vi "Launcher.vi"   [LabVIEW 2020]
uses:
  Executive/Executive/Executive.lvclass
  C:/Program Files (x86)/National Instruments/LabVIEW 2020/vi.lib/ActorFramework/Actor/Actor.lvclass
  <vilib>/ActorFramework/Actor/Actor.lvclass
panel:
  # "open_cst"
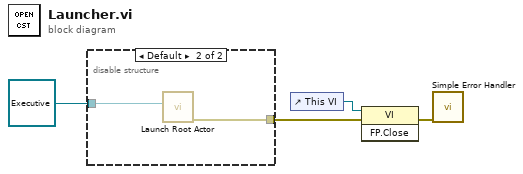
[diagram p0: block diagram]
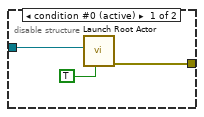
[diagram p2: hidden frame]
diagram:
  n1 = disable-structure shown="Default" {
    disable-tunnel: refnum<class "Executive.lvclass"> refnum ("Executive.lvlib:Executive.lvclass") -> [w7 w9]
    disable-tunnel: [w6 w8] -> w2
    frame condition #0 (active) {
      n2 = call <vilib>:"Launch Root Actor.vi"("Open Actor Core front panel? (F)"=TRUE, "Actor"=w7) -> ("error out"=w6:errorcluster)  [unwired: 8 in, 1 out]
    }
    frame condition #1 {
      n3 = call <vilib>:"Launch Root Actor.vi"("Actor"=w9) -> ("error out"=w8:errorcluster)  [unwired: 9 in, 1 out]
    }
  }
  n4 = control-ref of="This VI"() -> (w4:refnum<vi>)
  n5 = invoke class="VI" method="FP.Close"(reference=w4, error in=w2) -> (error out=w3:errorcluster)  [unwired: 1 in, 2 out]
  n6 = call <vilib>:"Simple Error Handler.vi"("error in (no error)"=w3) -> ()  [unwired: 4 in, 5 out]
